vi "FringeTrackerCalibrateRatio2.vi"(2 "Seconds":i32, 3 "FringeTracker Name":string="TipTiltMirror[1]", 9 "error in (no error)":errorcluster) -> (0 "FringeTracker Name out":string, 6 "error out":errorcluster caption="error in (no error)")   [LabVIEW 2009]
uses:
  lib/lvrtc.dll
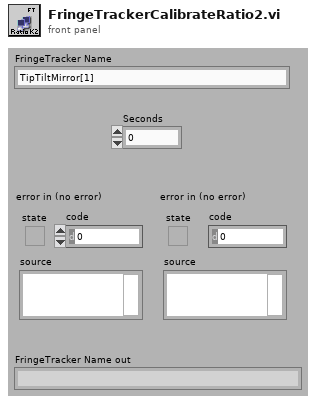
[diagram p1: front panel]
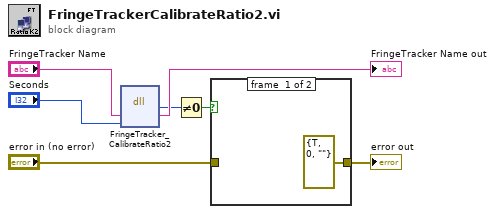
[diagram p0: block diagram]
diagram:
  n1 = dll-call lib="C:/Ohana/LV2009/OhanaOS-LV81/Instruments/RTC/Api/lib/lvrtc.dll" fn="FringeTracker_CalibrateRatio2"("FringeTrackerName"="FringeTracker Name", "seconds"="Seconds") -> ("return type"=w4:i32, "FringeTrackerName"=→"FringeTracker Name out":string)  [unwired: 4 in, 2 out]
  n2 = Not Equal To 0?(x=w4) -> (x != 0?=w3:bool)
  n3 = case shown="False" w3 {
    tunnel: "error in (no error)" -> [_ w9]
    tunnel: [errorcluster {"status"=TRUE, "code"=0, "source"=""} ("error in (no error)") w9] -> w2
    frame #0 {
    }
    frame #1 {
    }
  }
  "error out" <- w2
